vi "hmi_drivetrain.vi"(11 "UserData":T1) -> ()   [LabVIEW 2011]
uses:
  user_data.ctl
  user_buttons_dualaction.ctl
  user_buttons_360.ctl
  drivetrain/drivetrain_drive_write_thread.ctl
  drivetrain/gear_shift_state.ctl
  drivetrain/drivetrain_globals.vi
panel:
  in  "wheel filter const low":dbl=100.0
  in  "throttle filter const low":dbl=100.0
  in  "wheel filter const high":dbl=60.0
  in  "throttle filter const high":dbl=33.0
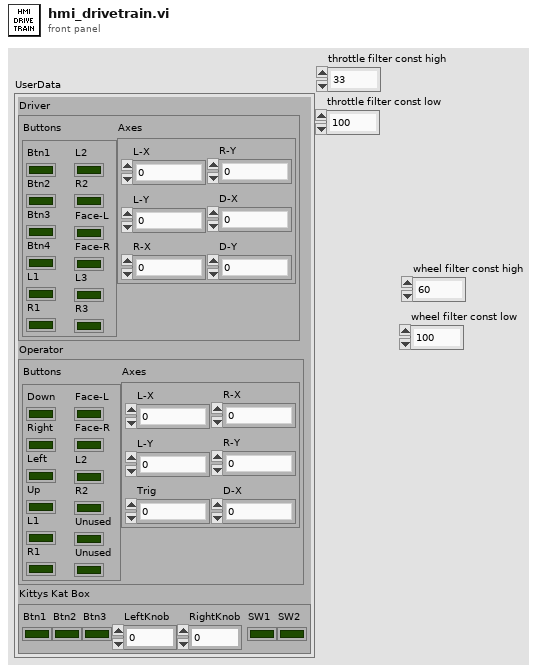
[diagram p1: front panel]
types:
  T1 = typedef "user_data.ctl" = cluster{"Driver":cluster{"Buttons":T2, "Axes":cluster{"L-X":dbl, "L-Y":dbl, "R-X":dbl, "R-Y":dbl, "D-X":dbl, "D-Y":dbl}}, "Operator":cluster{"Buttons":T3, "Axes":cluster{"L-X":dbl, "L-Y":dbl, "Trig":dbl, "R-X":dbl, "R-Y":dbl, "D-X":dbl}}, "Kittys Kat Box":cluster{"Btn1":bool, "Btn2":bool, "Btn3":bool, "LeftKnob":dbl, "RightKnob":dbl, "SW1":bool, "SW2":bool}}
  T2 = typedef "user_buttons_dualaction.ctl" = cluster{"Btn1":bool, "Btn2":bool, "Btn3":bool, "Btn4":bool, "L1":bool, "R1":bool, "L2":bool, "R2":bool, "Face-L":bool, "Face-R":bool, "L3":bool, "R3":bool}
  T3 = typedef "user_buttons_360.ctl" = cluster{"Down":bool, "Right":bool, "Left":bool, "Up":bool, "L1":bool, "R1":bool, "Face-L":bool, "Face-R":bool, "L2":bool, "R2":bool, "Unused":bool, "Unused":bool}
  T4 = typedef "gear_shift_state.ctl" = enum16{"low", "high"}
  T5 = typedef "drivetrain_drive_write_thread.ctl" = enum16{"Teleop", "Script Engine - Autonomous", "Script Engine - Sequence"}
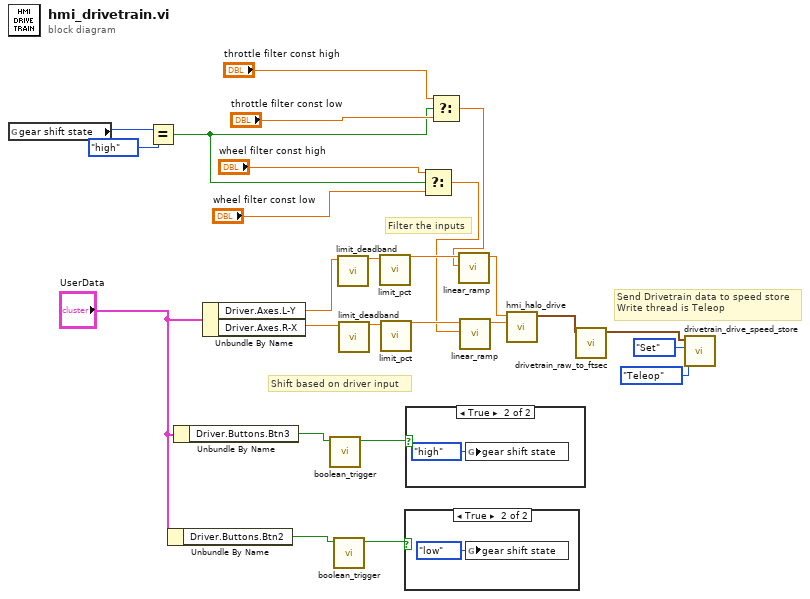
[diagram p0: block diagram]
diagram:
  # "Send Drivetrain data to speed store\nWrite thread is Teleop"
  # "Filter the inputs"
  # "Shift based on driver input"
  n1 = global read "drivetrain_globals.vi" "gear shift state"() -> (w8:T4)
  n2 = Equal?(x=w8, y=gear_shift_state."high") -> (x = y?=w2:bool)
  n3 = Unbundle By Name("UserData") -> ("Driver.Buttons.Btn2"=w19:bool)
  n4 = Unbundle By Name("UserData") -> ("Driver.Buttons.Btn3"=w21:bool)
  n5 = Unbundle By Name("UserData") -> ("Driver.Axes.L-Y"=w17:dbl, "Driver.Axes.R-X"=w11:dbl)
  n6 = call "boolean_trigger.vi"("Input"=w21) -> ("Rising Edge"=w20:bool)  [unwired: 10 in]
  n7 = call "boolean_trigger.vi"("Input"=w19) -> ("Rising Edge"=w18:bool)  [unwired: 10 in]
  n8 = call "limit_deadband.vi"("Val"=w17) -> ("Val Out"=w16:dbl)  [unwired: 10 in]
  n9 = call "limit_deadband.vi"("Val"=w11) -> ("Val Out"=w13:dbl)  [unwired: 10 in]
  n10 = call "limit_pct.vi"("PCT"=w16) -> ("PCT Out"=w15:dbl)  [unwired: 10 in]
  n11 = call "limit_pct.vi"("PCT"=w13) -> ("PCT Out"=w12:dbl)  [unwired: 10 in]
  n12 = case shown="True" w18 {
    frame False {
    }
    frame True {
      n13 = global write "drivetrain_globals.vi" "gear shift state"(gear_shift_state."low" ("gear shift state")) -> ()
    }
  }
  n14 = case shown="True" w20 {
    frame False {
    }
    frame True {
      n15 = global write "drivetrain_globals.vi" "gear shift state"(gear_shift_state."high" ("gear shift state")) -> ()
    }
  }
  n16 = Select(t="wheel filter const high", s=w2, f="wheel filter const low") -> (s? t:f=w4:dbl)
  n17 = Select(t="throttle filter const high", s=w2, f="throttle filter const low") -> (s? t:f=w6:dbl)
  n18 = call "linear_ramp.vi"("filter const (dx/dt)"=w6, "input"=w15) -> ("output"=w14:dbl)  [unwired: 9 in]
  n19 = call "linear_ramp.vi"("filter const (dx/dt)"=w4, "input"=w12) -> ("output"=w10:dbl)  [unwired: 9 in]
  n20 = call "hmi_halo_drive.vi"("Wheel"=w10, "Throttle"=w14) -> ("Drive Data"=w24:cluster{"Left":dbl, "Right":dbl})  [unwired: 9 in]
  n21 = call "drivetrain_raw_to_ftsec.vi"("Drive Data"=w24) -> ("Drive Data Out"=w25:cluster{"Left":dbl, "Right":dbl})  [unwired: 10 in]
  n22 = call "drivetrain_drive_speed_store.vi"("Write Thread"=drivetrain_drive_write_thread."Teleop", "data_store_mode"=enum16{"Set", "Get"}."Set", "drive data"=w25) -> ()  [unwired: 7 in, 2 out]
